vi "AIT 664 - ReadWrite Message.vi"(0 "Message In":T6={"Name"="", "xmlName"="", "Tx-Rx_T-Tx"=FALSE, "RT_Address"=0, "RT_SA_Address"=0, "Block Data Refs"=[], "Values Array"=[], "Length"=0, "Words"=0, "FIFO Index"=0, "RX Word"=0, "IterationOffset"=0, "Default Msg Data"=[], "Driver Data"={"First Word"=[], "Start Bit"=[], "Num Bits"=[], "Decimation"=0, "IterationOffset"=0, "Signed?"=[], "ScaleFac"=[], "ScaleOffset"=[]}, "Status Data"=[], "Queue Transmit Channel"=18446744073709551615, "Transmit Channel Data Reference"=0} {"Transmit Channel Data Reference" format="%.0x"; "Queue Transmit Channel" format="%.0x"; "Driver Data"."Num Bits" min=1 max=32; "Block Data Refs"."Data Reference" format="%.0x"}, 1 "Iteration":i32, 3 "Mode":T13, 5 "FIFOs In":T5, 7 "Channel Index":i32, 9 "Sampling Type":T1, 11 "error in (no error)":errorcluster, 12 "Tx Com Udp Port":T2 {"Handle" format="%08x"}) -> (4 "Message Out":T6={"Name"="", "xmlName"="", "Tx-Rx_T-Tx"=FALSE, "RT_Address"=0, "RT_SA_Address"=0, "Block Data Refs"=[], "Values Array"=[], "Length"=0, "Words"=0, "FIFO Index"=0, "RX Word"=0, "IterationOffset"=0, "Default Msg Data"=[], "Driver Data"={"First Word"=[], "Start Bit"=[], "Num Bits"=[], "Decimation"=0, "IterationOffset"=0, "Signed?"=[], "ScaleFac"=[], "ScaleOffset"=[]}, "Status Data"=[], "Queue Transmit Channel"=18446744073709551615, "Transmit Channel Data Reference"=0} {"Transmit Channel Data Reference" format="%.0x"; "Queue Transmit Channel" format="%.0x"; "Driver Data"."Num Bits" min=1 max=32; "Block Data Refs"."Data Reference" format="%.0x"}, 6 "FIFOs Out":T5, 14 "Tx Com Udp Port out":T2 {"Handle" format="%08x"}, 15 "error out":errorcluster)   [LabVIEW 2015, in "AIT 664 Custom Device.lvlib"]
doc: "Read/Write hardware, Read/Write veristand data"
uses:
  AIT 664 Custom Device.lvlib
  RT Controls/ReadWrite Selector.ctl
  RT Controls/AIT 664 - RT Message Settings.ctl
  <vilib>/NI Veristand/Custom Device API/Block Data Reference.ctl
  <vilib>/NI Veristand/Custom Device API/Data Reference.ctl
  RT Controls/AIT 664 - Driver Data.ctl
  Controls and Global/Start Bit.ctl
  Controls and Global/Number of Bits.ctl
  <vilib>/NI Veristand/Custom Device API/Custom Device Item Ref.ctl
  RT Controls/FIFO.ctl
  <userlib>/ARINC 664/AIT 664 Controls/General/Message Port.ctl
  <userlib>/ARINC 664/AIT 664 Controls/General/Direction.ctl
  <userlib>/ARINC 664/AIT 664 Controls/General/Message Port Type.ctl
  System Explorer/Controls/664 - Sampling Type.ctl
  <vilib>/NI Veristand/Custom Device API/Global Data Refs.vi
  <vilib>/NI Veristand/Custom Device API/Custom Device API.lvlib
  <userlib>/ARINC 664/AIT 664 API.lvlib
panel:
  out "Sampling Type out":T1
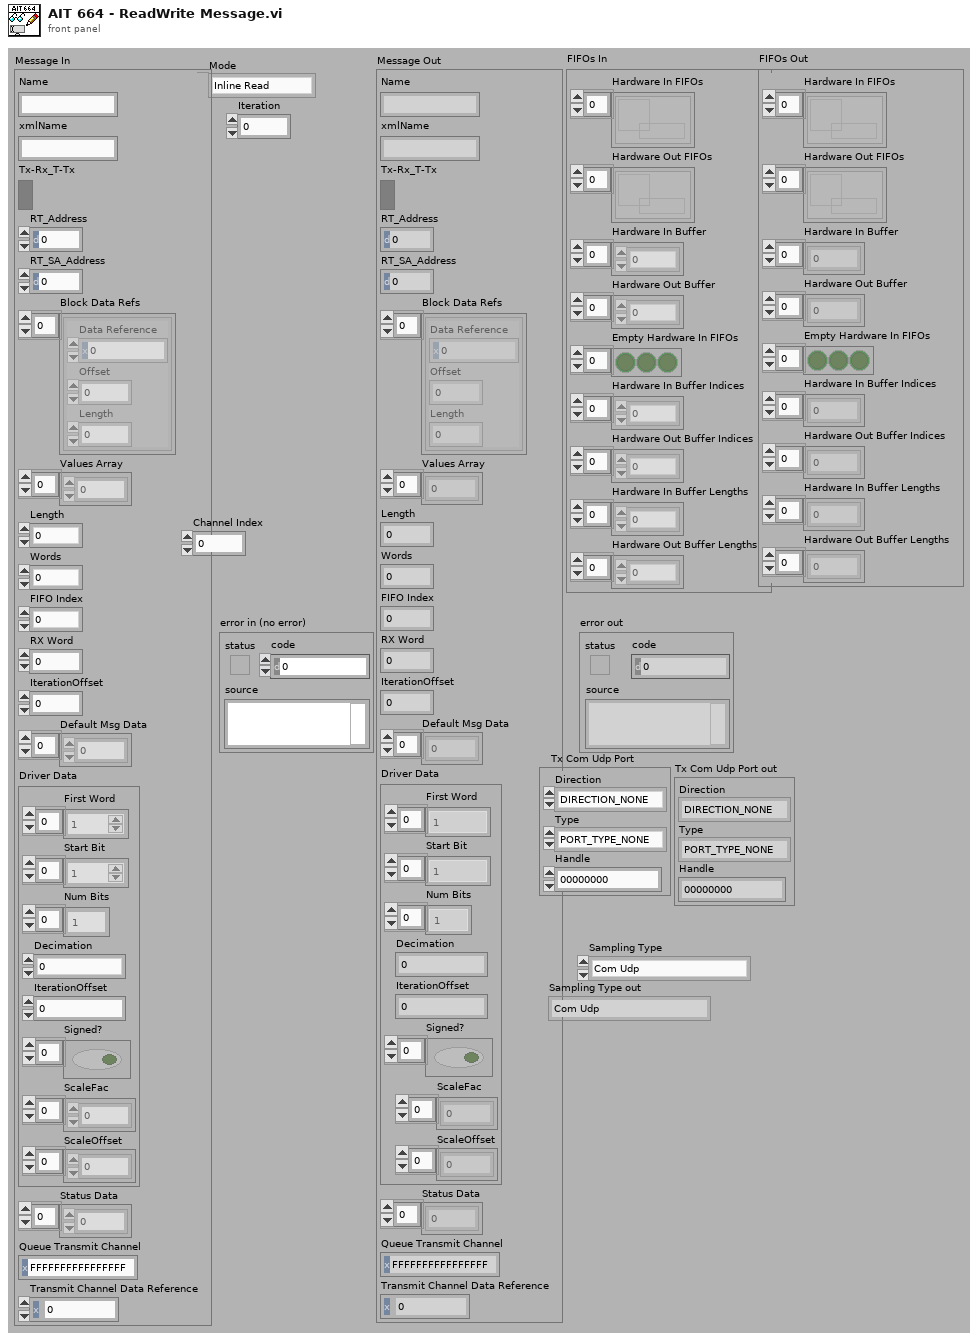
[diagram p1: front panel]
types:
  T1 = typedef "AIT 664 Custom Device.lvlib/664 - Sampling Type.ctl" = enum16{"Com Udp", "Com Udp Queuing", "Sap Udp", "Sap Ip", "Sap Mac", "Unknown"}
  T2 = typedef "AIT 664 API.lvlib/Message Port.ctl" = cluster{"Direction":T3, "Type":T4, "Handle":u64}
  T3 = typedef "AIT 664 API.lvlib/Direction.ctl" = enum16{"DIRECTION_NONE", "DIRECTION_TX", "DIRECTION_RX"}
  T4 = typedef "AIT 664 API.lvlib/Message Port Type.ctl" = enum16{"PORT_TYPE_NONE", "COM_UDP", "SAP_UDP", "SAP_IP", "SAP_MAC", "COTS_MAC", "COTS_MAC_RAW"}
  T5 = typedef "AIT 664 Custom Device.lvlib/FIFO.ctl" = cluster{"Hardware In FIFOs":refnum<k33>[], "Hardware Out FIFOs":refnum<k33>[], "Hardware In Buffer":dbl[], "Hardware Out Buffer":dbl[], "Empty Hardware In FIFOs":bool[], "Hardware In Buffer Indices":i32[], "Hardware Out Buffer Indices":i32[], "Hardware In Buffer Lengths":i32[], "Hardware Out Buffer Lengths":i32[]}
  T6 = typedef "AIT 664 Custom Device.lvlib/AIT 664 - RT Message Settings.ctl" = cluster{"Name":string, "xmlName":string, "Tx-Rx_T-Tx":bool, "RT_Address":u8, "RT_SA_Address":u8, "Block Data Refs":T7[], "Values Array":dbl[], "Length":i32, "Words":i32, "FIFO Index":i32, "RX Word":u32, "IterationOffset":i32, "Default Msg Data":u8[], "Driver Data":T9, "Status Data":u32[], "Queue Transmit Channel":T12, "Transmit Channel Data Reference":T8}
  T7 = typedef "Custom Device API.lvlib/Block Data Reference.ctl" = cluster{"Data Reference":T8, "Offset":u64, "Length":u64}
  T8 = typedef "Custom Device API.lvlib/Data Reference.ctl" = i32
  T9 = typedef "AIT 664 Custom Device.lvlib/AIT 664 - Driver Data.ctl" = cluster{"First Word":T10[], "Start Bit":T10[], "Num Bits":T11[], "Decimation":i32, "IterationOffset":i32, "Signed?":bool[], "ScaleFac":dbl[], "ScaleOffset":dbl[]}
  T10 = typedef "AIT 664 Custom Device.lvlib/Start Bit.ctl" = i32
  T11 = typedef "AIT 664 Custom Device.lvlib/Number of Bits.ctl" = i32
  T12 = typedef "Custom Device API.lvlib/Custom Device Item Ref.ctl" = u64
  T13 = typedef "AIT 664 Custom Device.lvlib/ReadWrite Selector.ctl" = enum16{"Inline Read", "Inline Write", "Async HWIn", "Async HWOut"}
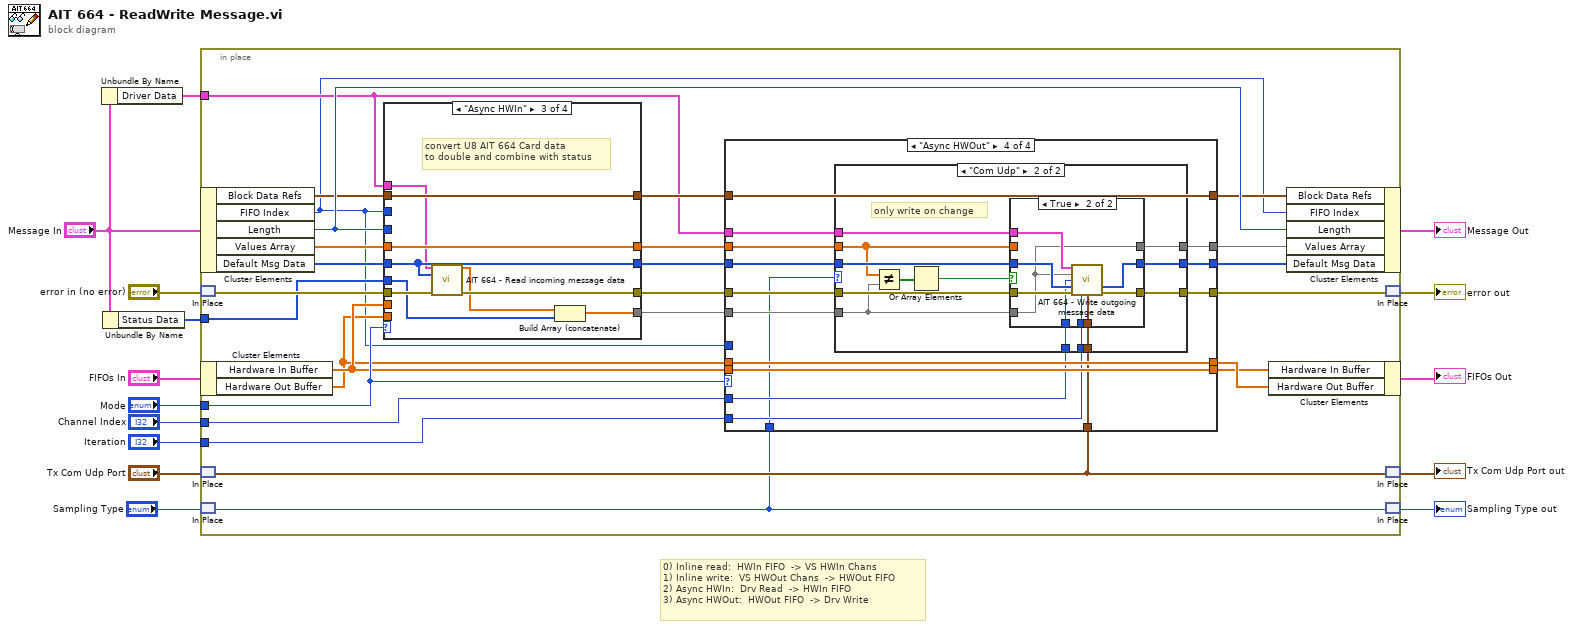
[diagram p0: block diagram]
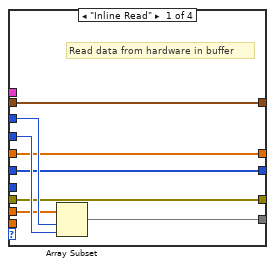
[diagram p2: hidden frame]
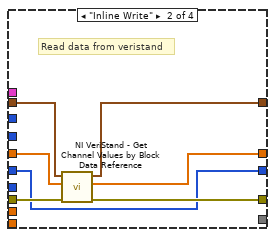
[diagram p3: hidden frame]
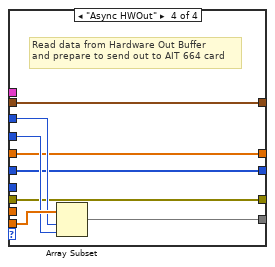
[diagram p4: hidden frame]
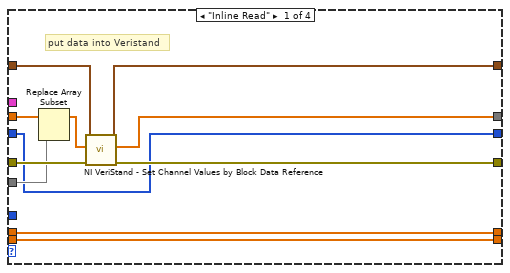
[diagram p5: hidden frame]
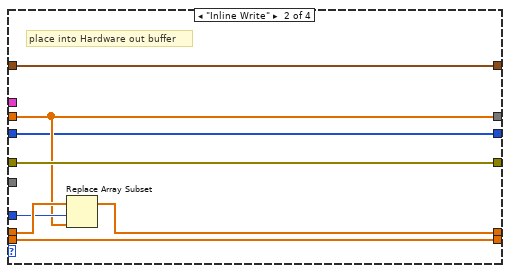
[diagram p6: hidden frame]
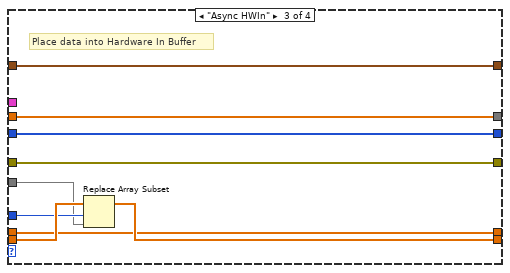
[diagram p7: hidden frame]
diagram:
  # "0) Inline read:\t\tHWIn FIFO \t-> VS HWIn Chans\n1) Inline write: \tVS HWOut Chans \t-> HWOut FIFO\n2) Async HWIn:\t\tDrv Read \t-> HWIn FIFO\n3) Async HWOut: \tHWOut FIFO \t-> Drv Write"
  n1 = Unbundle By Name("Message In") -> ("Driver Data"=w8:T9)
  n2 = Unbundle By Name("Message In") -> ("Status Data"=w6:u32[])
  n3 = in-place {
    in-place-border: "Mode" -> [w27]
    in-place-border: "Iteration" -> [w31]
    in-place-border: "Channel Index" -> [w18]
    in-place-border: w8 -> [w21]
    in-place-border: w6 -> [w20]
    n4 = in-place-cluster #1("Message In") -> ("Block Data Refs"=w25:T7[], "FIFO Index"=w16:i32, "Length"=w39:i32, "Values Array"=w36:dbl[], "Default Msg Data"=w30:u8[])
    n5 = in-place-match #2("error in (no error)") -> (w38:errorcluster)
    n6 = in-place-cluster #3("FIFOs In") -> ("Hardware In Buffer"=w23:dbl[], "Hardware Out Buffer"=w22:dbl[])
    n7 = in-place-match #4("Tx Com Udp Port") -> (w19:T2)
    n8 = in-place-match #5("Sampling Type") -> (w17:T1)
    n9 = case shown="\"Async HWIn\"" w27 {
      tunnel: w23 -> [w47 _ _ _]
      tunnel: w16 -> [w49 _ _ w72]
      tunnel: w39 -> [w48 _ _ w71]
      tunnel: [w43 _ w58 w67] -> w41
      tunnel: w38 -> [w45 w56 w63 w68]
      tunnel: [w45 w55 w62 w68] -> w37
      tunnel: w25 -> [w46 w54 w65 w69]
      tunnel: w36 -> [w42 w53 w64 w70]
      tunnel: [w42 w52 w64 w70] -> w34
      tunnel: [w46 w51 w65 w69] -> w35
      tunnel: w21 -> [_ _ w60 _]
      tunnel: w22 -> [_ _ _ w73]
      tunnel: w30 -> [w44 w50 w61 w66]
      tunnel: [w44 w50 w61 w66] -> w29
      tunnel: w20 -> [_ _ w57 _]
      frame "Inline Read" {
        # "Read data from hardware in buffer"
        n10 = Array Subset(array=w47, index=w49, length=w48) -> (w43:dbl[])
      }
      frame "Inline Write" {
        # "Read data from veristand"
        n11 = call <vilib>:"NI VeriStand - Get Channel Values by Block Data Reference.vi"("error in (no error)"=w56, "Values Array in"=w53, "Block Data Ref"=w54) -> ("error out"=w55:errorcluster, "Values Array out"=w52:dbl[], "Block Data Ref dup"=w51:T7[])  [unwired: 6 in]
      }
      frame "Async HWIn" {
        # "convert U8 AIT 664 Card data\nto double and combine with status"
        n12 = call "AIT 664 - Read incoming message data.vi"("Driver Data"=w60, "Default Msg Data"=w61, "error in (no error)"=w63) -> ("Values"=w59:dbl[], "error out"=w62:errorcluster)  [unwired: 11 in]
        n13 = Build Array (concatenate)(w59, w57) -> (w58:dbl[])
      }
      frame "Async HWOut" {
        # "Read data from Hardware Out Buffer\nand prepare to send out to AIT 664 card"
        n14 = Array Subset(array=w73, index=w72, length=w71) -> (w67:dbl[])
      }
    }
    n15 = case shown="\"Async HWOut\"" w27 {
      tunnel: w35 -> [w78 w89 w101 w114]
      tunnel: w41 -> [w82 _ w94 w106]
      tunnel: w37 -> [w84 w90 w97 w113]
      tunnel: [w83 w90 w97 w112] -> w40
      tunnel: w34 -> [w77 w88 w95 w104]
      tunnel: [w75 w88 w95 w103] -> w26
      tunnel: [w81 w89 w101 w114] -> w24
      tunnel: w22 -> [w80 w92 w96 w115]
      tunnel: [w80 w85 w96 w115] -> w33
      tunnel: w16 -> [_ w91 w98 _]
      tunnel: w23 -> [w79 w87 w100 w116]
      tunnel: [w79 w87 w99 w116] -> w32
      tunnel: w21 -> [_ _ _ w105]
      tunnel: w31 -> [_ _ _ w108]
      tunnel: w29 -> [w76 w86 w93 w111]
      tunnel: [w76 w86 w93 w110] -> w28
      tunnel: w18 -> [_ _ _ w109]
      tunnel: w19 -> [_ _ _ w107]
      tunnel: w17 -> [_ _ _ w102]
      frame "Inline Read" {
        # "put data into Veristand"
        n16 = Replace Array Subset(array=w77, new element=w82) -> (w74:dbl[])  [unwired: 1 in]
        n17 = call <vilib>:"NI VeriStand - Set Channel Values by Block Data Reference.vi"("error in (no error)"=w84, "Values Array in"=w74, "Block Data Ref"=w78) -> ("error out"=w83:errorcluster, "Values Array out"=w75:dbl[], "Block Data Ref dup"=w81:T7[])  [unwired: 6 in]
      }
      frame "Inline Write" {
        # "place into Hardware out buffer"
        n18 = Replace Array Subset(array=w92, new element=w88, index=w91) -> (w85:dbl[])
      }
      frame "Async HWIn" {
        # "Place data into Hardware In Buffer"
        n19 = Replace Array Subset(array=w100, new element=w94, index=w98) -> (w99:dbl[])
      }
      frame "Async HWOut" {
        n20 = case shown="\"Com Udp\"" w102 {
          tunnel: w113 -> [w117 w132]
          tunnel: [w117 w131] -> w112
          tunnel: w111 -> [w118 w130]
          tunnel: [w118 w129] -> w110
          tunnel: w109 -> [_ w128]
          tunnel: w108 -> [_ w127]
          tunnel: w107 -> [_ w126]
          tunnel: w106 -> [_ w124]
          tunnel: w105 -> [_ w125]
          tunnel: w104 -> [w119 w121]
          tunnel: [w119 w120] -> w103
          frame "Com Udp Queuing", Default {
            # "Since this is triggered by the user\ntransmit is done in the pcl,\ncannot access veristand channels in async loop"
          }
          frame "Com Udp" {
            # "only write on change"
            n21 = Not Equal?(x=w121, y=w124) -> (x != y?=w122:bool[])
            n22 = Or Array Elements(Boolean array=w122) -> (logical OR=w123:bool)
            n23 = case shown="True" w123 {
              tunnel: w132 -> [w133 w144]
              tunnel: [w133 w143] -> w131
              tunnel: w130 -> [w134 w142]
              tunnel: [w134 w141] -> w129
              tunnel: w128 -> [_ w140]
              tunnel: w127 -> [_ w139]
              tunnel: w126 -> [_ w138]
              tunnel: w125 -> [_ w137]
              tunnel: w124 -> [_ w136]
              tunnel: w121 -> [w135 _]
              tunnel: [w135 w136] -> w120
              frame False {
              }
              frame True {
                n24 = call "AIT 664 - Write outgoing message data.vi"("Driver Data"=w137, "Values"=w136, "Channel Index"=w140, "Msg Data In"=w142, "error in (no error)"=w144, "Iteration"=w139, "Tx Com Udp Port"=w138) -> ("Msg Data Out"=w141:u8[], "error out"=w143:errorcluster)  [unwired: 7 in]
              }
            }
          }
        }
      }
    }
    n25 = in-place-cluster #3("Hardware In Buffer"=w32, "Hardware Out Buffer"=w33) -> (→"FIFOs Out":T5)
    n26 = in-place-cluster #1("Block Data Refs"=w24, "FIFO Index"=w16, "Length"=w39, "Values Array"=w26, "Default Msg Data"=w28) -> (→"Message Out":T6)
    n27 = in-place-match #2(w40) -> (→"error out":errorcluster)
    n28 = in-place-match #4(w19) -> (→"Tx Com Udp Port out":T2)
    n29 = in-place-match #5(w17) -> (→"Sampling Type out":T1)
  }
